vi "Main.vi"() -> ()   [LabVIEW 2013]
uses:
  Ctl/ViewCtl.ctl
  USBCAN/DevType.ctl
  Ctl/DeviceCtl.ctl
  Ctl/ActionCtl.ctl
  Ctl/ResultCtl.ctl
  Ctl/Logctl.ctl
  Ctl/SinResult.ctl
  Global.vi
panel:
  out "Time":u32
  out "Log":refnum<user-event>
  in  "Log":T1
  out "Result":refnum<user-event>
  in  "Result":T2
  in  "输出簇":T3
  in  "设备":T4
  in  "结果显示":T5
  in  "退出":bool
  in  "选项卡控件":enum32{"运行界面", "参数配置", "帮助"}(tab)
  in  "测试方式":enum16{"震动前测试", "震动测试"}(ring)
  in  "设置":bool
  in  "急停":bool
  in  "启动":bool
  out "通信8显示":string
  out "通信7显示":string
  out "通信6显示":string
  out "通信5显示":string
  out "通信4显示":string
  out "通信3显示":string
  out "通信2显示":string
  out "通信1显示":string
  in  "CAN1":bool
  out "CAN1显示":bool
  out "CAN2显示":bool
  in  "CAN2":bool
  out "CAN3显示":bool
  in  "CAN3":bool
  out "CAN4显示":bool
  in  "CAN4":bool
  out "CAN5显示":bool
  in  "CAN5":bool
  out "CAN6显示":bool
  in  "CAN6":bool
  out "CAN7显示":bool
  in  "CAN7":bool
  out "CAN8显示":bool
  in  "CAN8":bool
  out "总结果显示":string
  out "当前模式":string
  in  "COM1":refnum<visa-resource-name>="COM62" caption="COM"
  in  "设备索引1":u16(ring) caption="索引" items=["0", "1", "2", "3", "4", "5", "6", "7"]
  in  "设备索引2":u16(ring)=1 caption="索引" items=["0", "1", "2", "3", "4", "5", "6", "7"]
  in  "COM2":refnum<visa-resource-name>="COM2" caption="COM"
  in  "设备索引3":u16(ring)=2 caption="索引" items=["0", "1", "2", "3", "4", "5", "6", "7"]
  in  "COM3":refnum<visa-resource-name>="COM3" caption="COM"
  in  "设备索引4":u16(ring)=3 caption="索引" items=["0", "1", "2", "3", "4", "5", "6", "7"]
  in  "COM4":refnum<visa-resource-name>="COM4" caption="COM"
  in  "设备索引5":u16(ring)=4 caption="索引" items=["0", "1", "2", "3", "4", "5", "6", "7"]
  in  "COM5":refnum<visa-resource-name>="COM5" caption="COM"
  in  "设备索引6":u16(ring)=5 caption="索引" items=["0", "1", "2", "3", "4", "5", "6", "7"]
  in  "COM6":refnum<visa-resource-name>="COM6" caption="COM"
  in  "设备索引7":u16(ring)=6 caption="索引" items=["0", "1", "2", "3", "4", "5", "6", "7"]
  in  "COM7":refnum<visa-resource-name>="COM7" caption="COM"
  in  "COM8":refnum<visa-resource-name>="COM8" caption="COM"
  in  "设备索引8":u16(ring)=7 caption="索引" items=["0", "1", "2", "3", "4", "5", "6", "7"]
  out "log":string
  out "参数":T7={"帧ID1"=0, "等待延时"=0, "间隔延时"=0, "总时间"=0, "总次数"=0, "发送数据1"="", "接收数据1"="", "发送数据2"="", "接收数据2"="", "CAN盒类型"=3, "帧ID2"=0, "同步启动个数"=8, "模式"=enum."整体", "Baud"=12} {"Baud" items=["250k bps"=10, "10k bps"=2, "5k bps"=1, "50k bps"=5, "40k bps"=4, "20k bps"=3, "80k bps"=6, "100k bps"=7, "125k bps"=8, "200k bps"=9, "400k bps"=11, "500k bps"=12, "666k bps"=13, "800k bps"=14, "1000k bps"=15]; "帧ID2" format="%.0x"; "CAN盒类型" items=["PCI-CAN200"=7, "USB-CAN"=2, "USB-CAN200"=3]; "帧ID1" format="%.0x"}
  # "帧ID\n发送数据域\n接收数据域\n等待延时\n间隔延时\n总次数\n总时间\nCAN盒类型下拉表\n模式：单盒分开测试、整体一起测试 \n布尔显示结果\n布尔开始按钮\n布尔总启动按钮\n过程字符串显示"
  # "ms"
  # "ms"
  # "s"
  # "ms"
  # "ms"
  # "s"
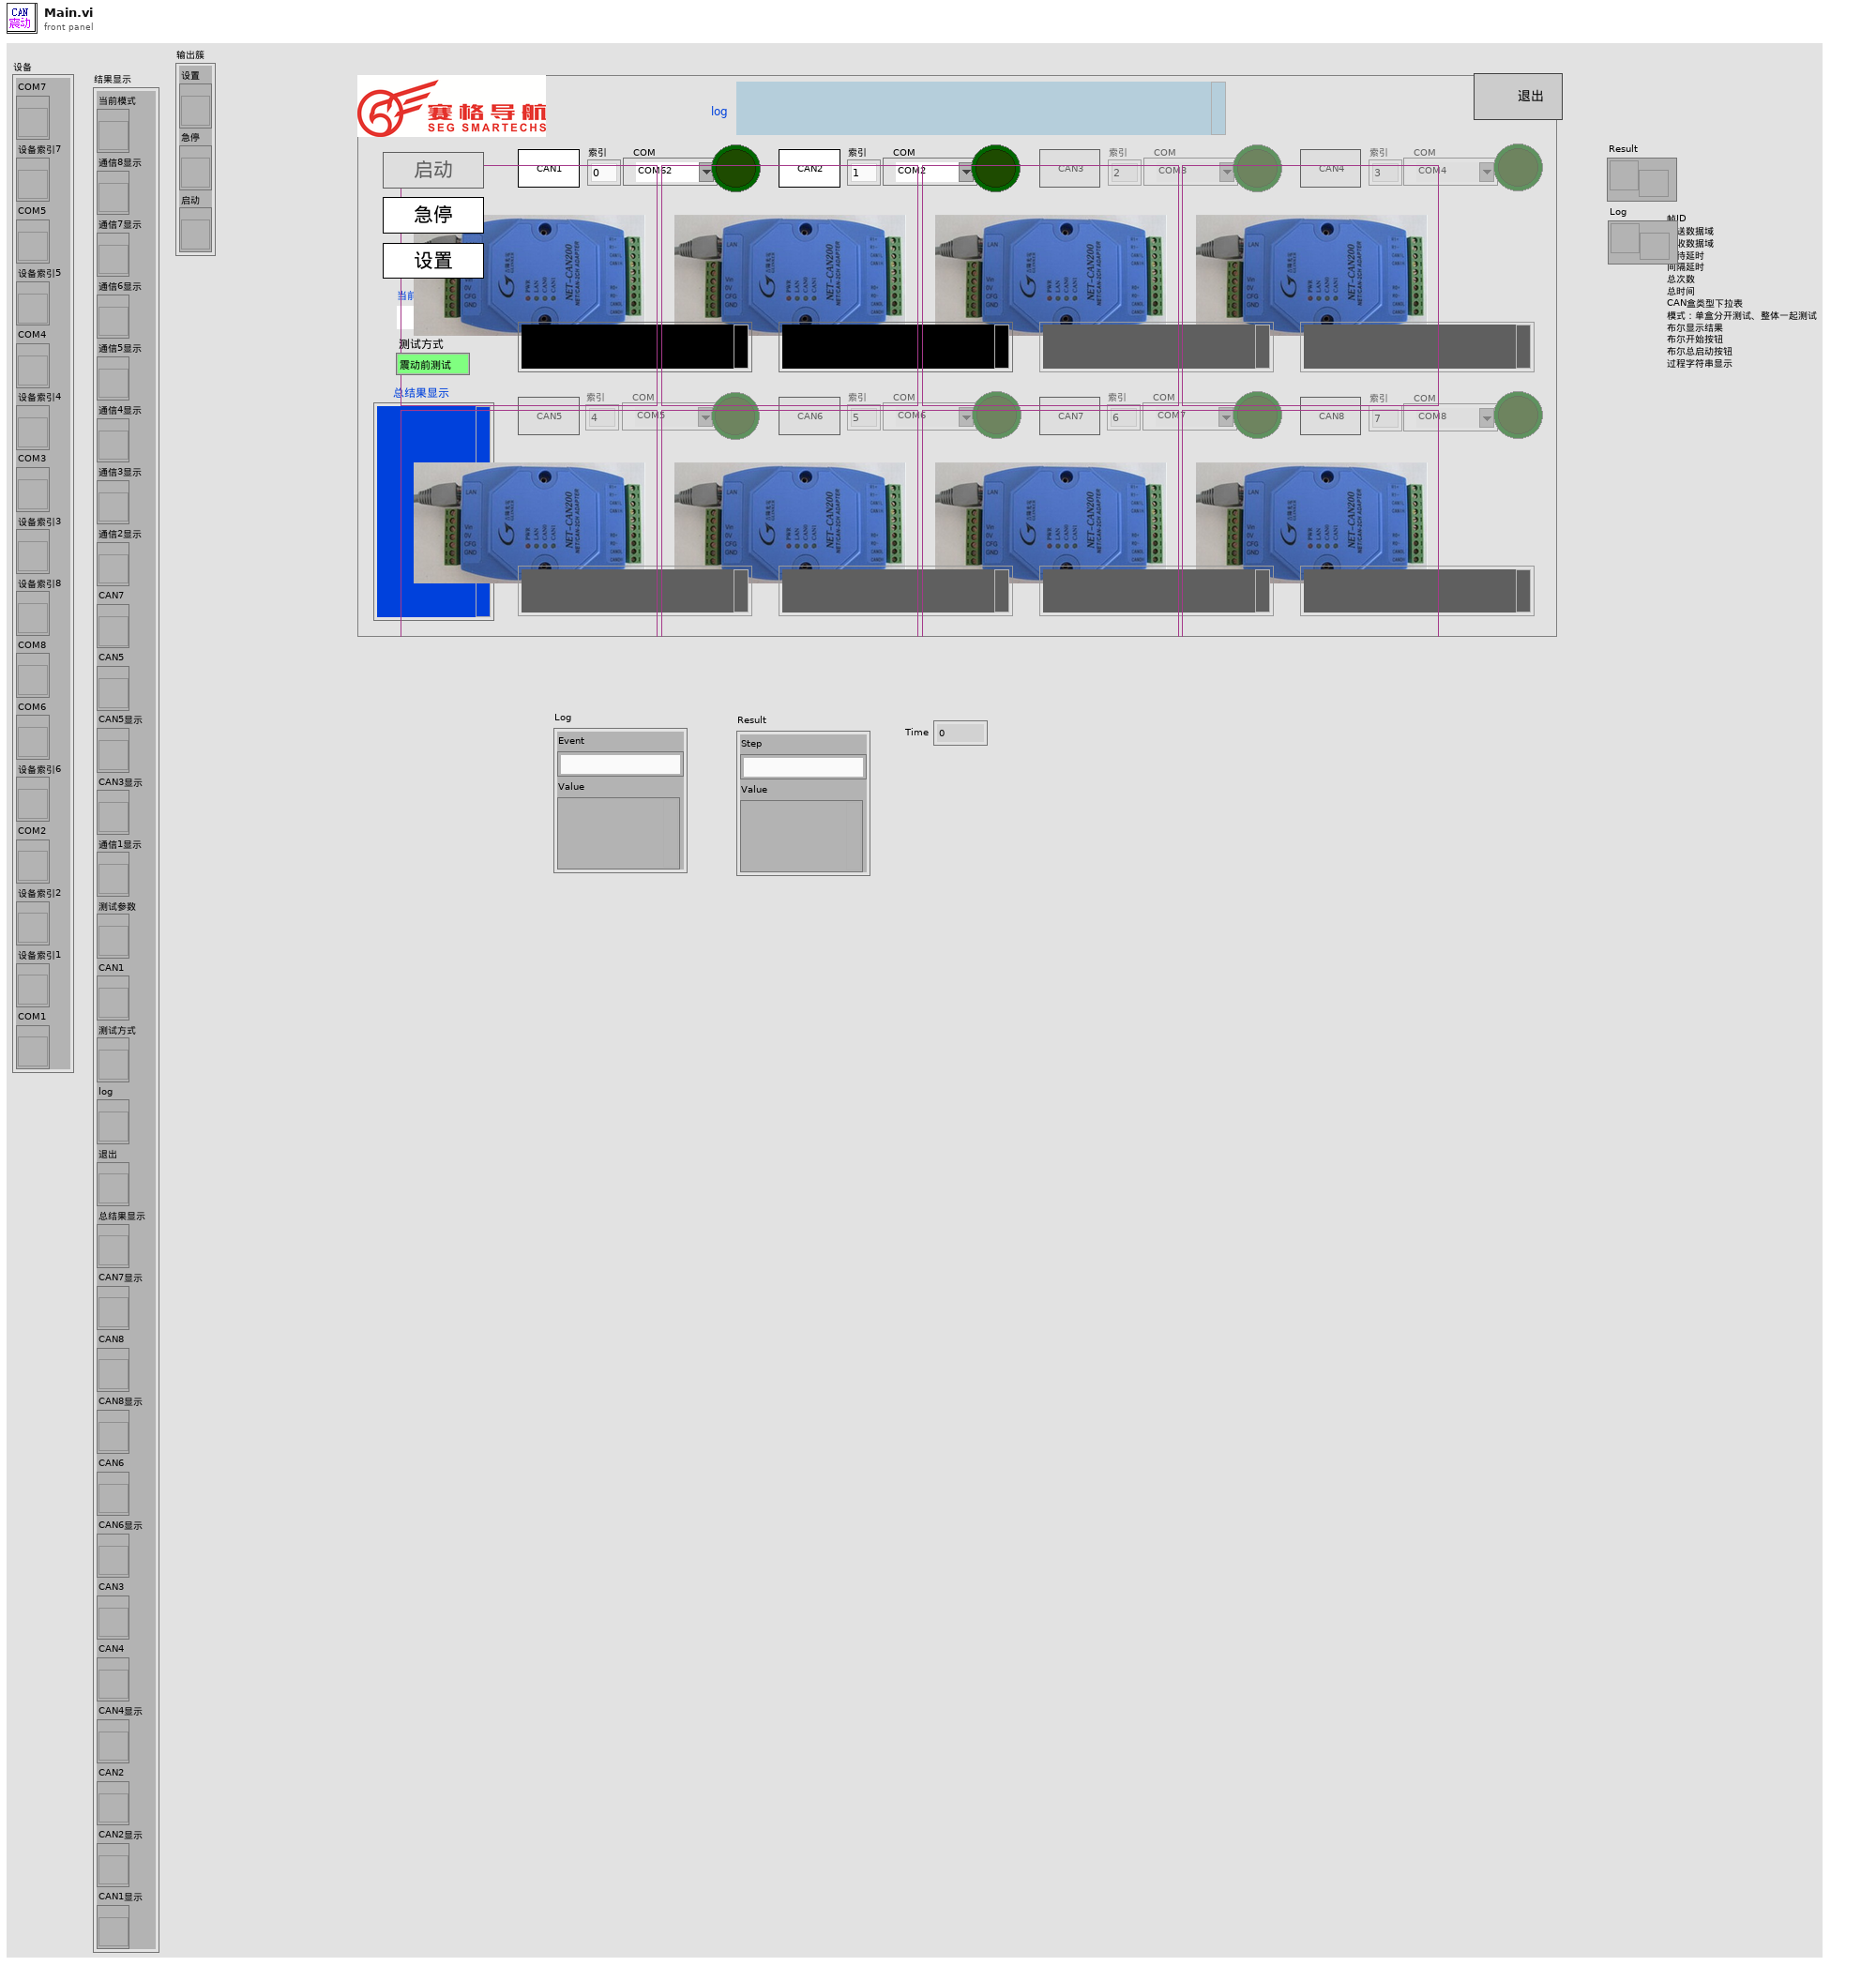
[diagram p1: front panel]
types:
  T1 = typedef "Logctl.ctl" = cluster{"Event":string, "Value":variant}
  T2 = typedef "ResultCtl.ctl" = cluster{"Step":string, "Value":variant}
  T3 = typedef "ActionCtl.ctl" = cluster{"设置":refnum<vi>, "急停":refnum<vi>, "启动":refnum<vi>}
  T4 = typedef "DeviceCtl.ctl" = cluster{"COM7":refnum<vi>, "设备索引7":refnum<vi>, "COM5":refnum<vi>, "设备索引5":refnum<vi>, "COM4":refnum<vi>, "设备索引4":refnum<vi>, "COM3":refnum<vi>, "设备索引3":refnum<vi>, "设备索引8":refnum<vi>, "COM8":refnum<vi>, "COM6":refnum<vi>, "设备索引6":refnum<vi>, "COM2":refnum<vi>, "设备索引2":refnum<vi>, "设备索引1":refnum<vi>, "COM1":refnum<vi>}
  T5 = typedef "ViewCtl.ctl" = cluster{"当前模式":refnum<vi>, "通信8显示":refnum<vi>, "通信7显示":refnum<vi>, "通信6显示":refnum<vi>, "通信5显示":refnum<vi>, "通信4显示":refnum<vi>, "通信3显示":refnum<vi>, "通信2显示":refnum<vi>, "CAN7":refnum<vi>, "CAN5":refnum<vi>, "CAN5显示":refnum<vi>, "CAN3显示":refnum<vi>, "通信1显示":refnum<vi>, "测试参数":refnum<vi>, "CAN1":refnum<vi>, "测试方式":refnum<vi>, "log":refnum<vi>, "退出":refnum<vi>, "总结果显示":refnum<vi>, "CAN7显示":refnum<vi>, "CAN8":refnum<vi>, "CAN8显示":refnum<vi>, "CAN6":refnum<vi>, "CAN6显示":refnum<vi>, "CAN3":refnum<vi>, "CAN4":refnum<vi>, "CAN4显示":refnum<vi>, "CAN2":refnum<vi>, "CAN2显示":refnum<vi>, "CAN1显示":refnum<vi>}
  T6 = typedef "DevType.ctl" = u16
  T7 = cluster{"帧ID1":u32, "等待延时":u32, "间隔延时":u32, "总时间":u32, "总次数":u32, "发送数据1":string, "接收数据1":string, "发送数据2":string, "接收数据2":string, "CAN盒类型":T6, "帧ID2":u32, "同步启动个数":u8, "模式":enum16{"整体", "单个"}, "Baud":u8}
  T8 = enum16{"CAN1", "CAN2", "CAN3", "CAN4", "CAN5", "CAN6", "CAN7", "CAN8"}
  T9 = enum16{"CAN1", "CAN2", "CAN3", "CAN4", "CAN5", "CAN6", "CAN7", "CAN8"}[]
  T10 = cluster{"事件注册引用句柄":refnum<event-registration>, "事件注册引用句柄":refnum<event-registration>}
  T11 = cluster{"COM1":refnum<visa-resource-name>, "COM2":refnum<visa-resource-name>, "COM3":refnum<visa-resource-name>, "COM4":refnum<visa-resource-name>, "COM5":refnum<visa-resource-name>, "COM6":refnum<visa-resource-name>, "COM7":refnum<visa-resource-name>, "COM8":refnum<visa-resource-name>}
  T12 = cluster{"帧ID1":bool, "等待延时":bool, "间隔延时":bool, "总时间":bool, "总次数":bool, "发送数据1":bool, "接收数据1":bool, "发送数据2":bool, "接收数据2":bool, "CAN盒类型":bool, "帧ID2":bool, "同步启动个数":bool, "模式":bool, "Baud":bool}
  T13 = typedef "SinResult.ctl" = cluster{"CAN通道":string, "TsRes":bool}
  T14 = cluster{"kCanBaud":u8, "DeviceType":T6, "DevInd":u16, "间隔延时":u32, "ID1(Hex)":string, "DataIN1(Hex)":string, "DataRec1(Hex)":string, "ID2(Hex)":string, "DataIN2(Hex)":string, "DataRec2(Hex)":string}
  T15 = enum32{"invalid app kind", "Development System", "Run Time System", "Student Edition", "Embedded LabVIEW", "Evaluation", "Custom"}
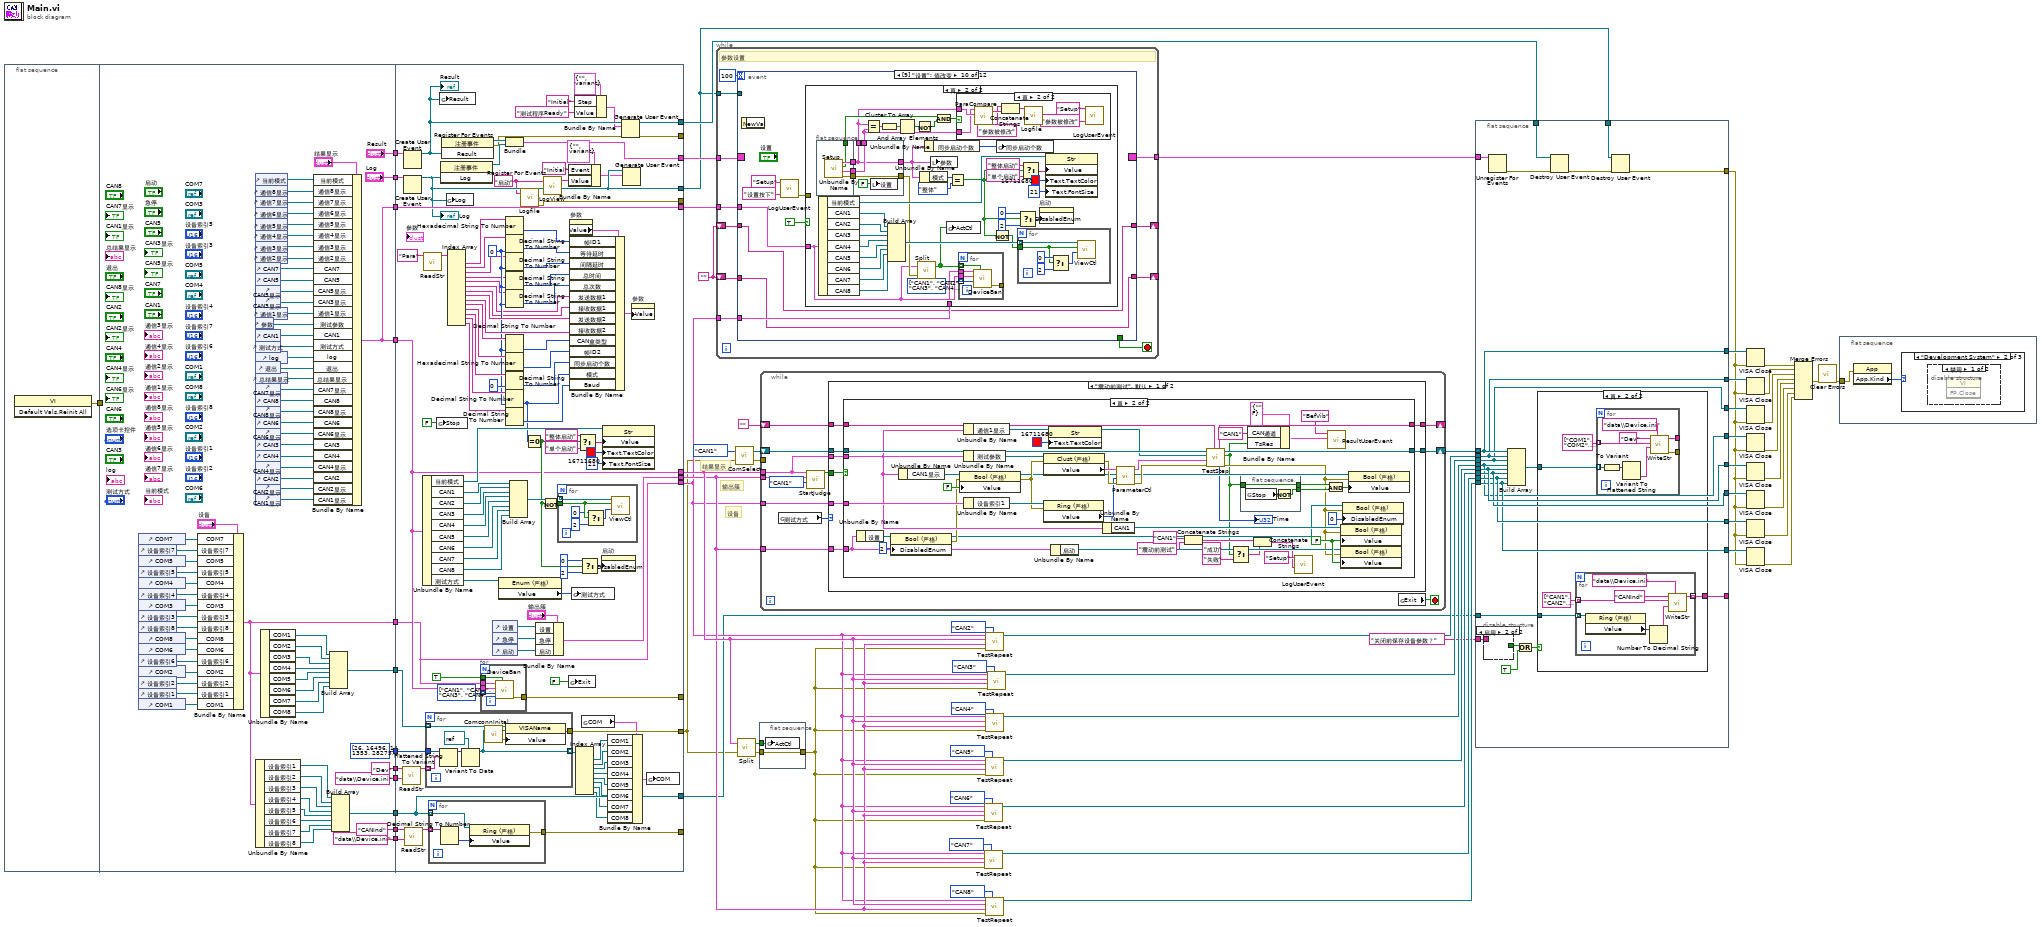
[diagram p0: block diagram]
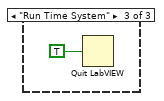
[diagram p4: hidden frame]
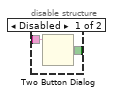
[diagram p5: hidden frame]
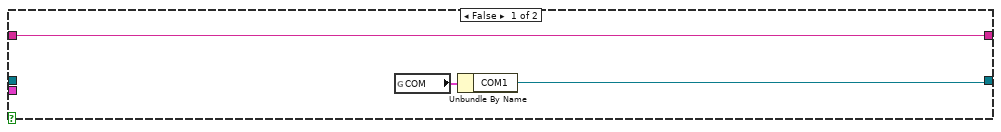
[diagram p7: hidden frame]
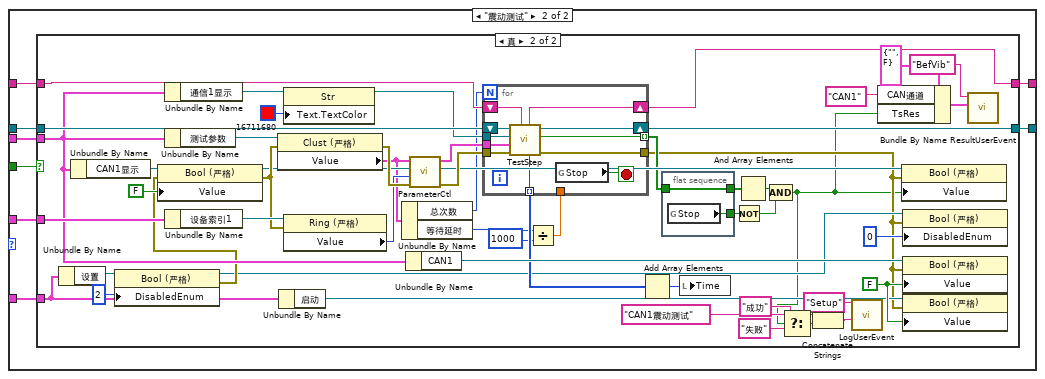
[diagram p8: hidden frame]
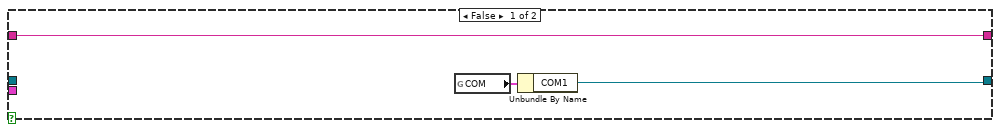
[diagram p9: hidden frame]
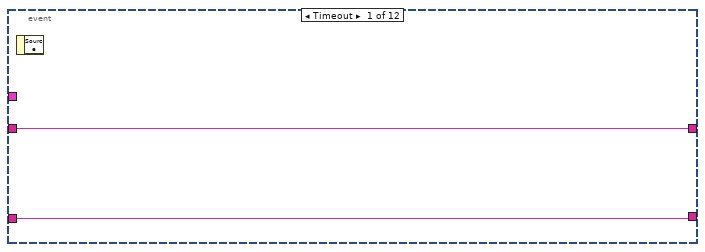
[diagram p10: hidden frame]
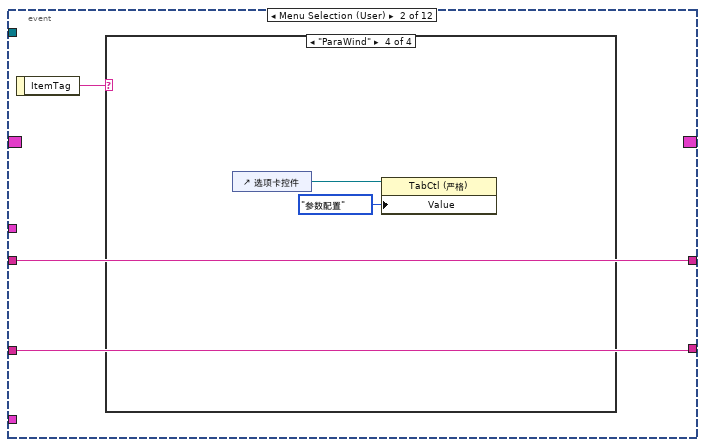
[diagram p11: hidden frame]
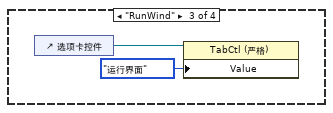
[diagram p14: hidden frame]
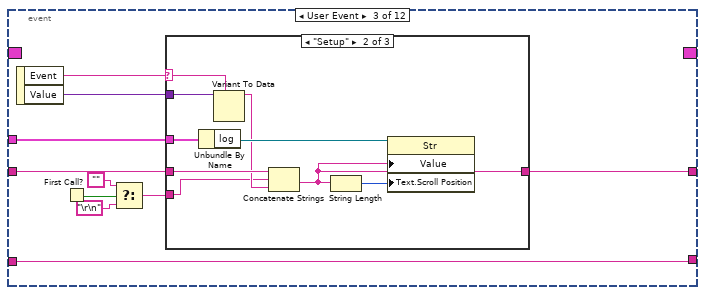
[diagram p15: hidden frame]
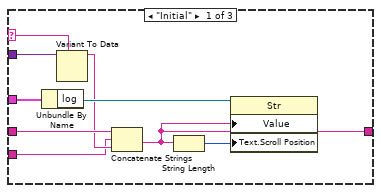
[diagram p16: hidden frame]
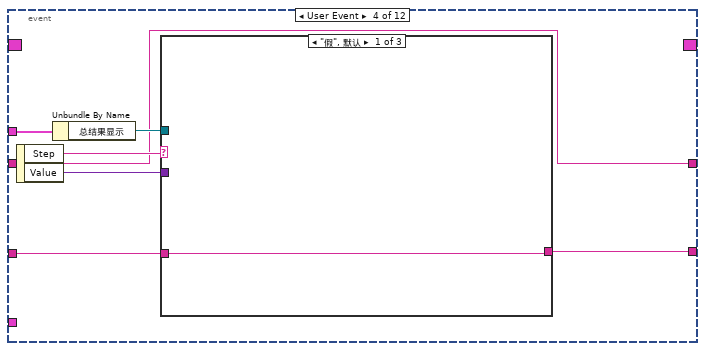
[diagram p18: hidden frame]
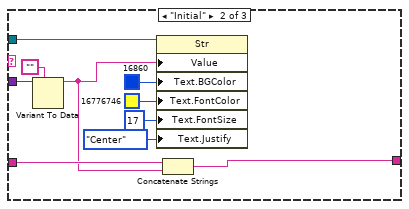
[diagram p19: hidden frame]
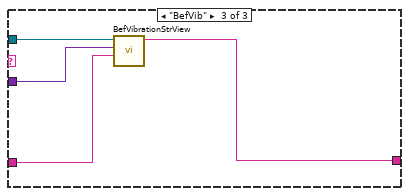
[diagram p20: hidden frame]
diagram:
  w26 = ""
  # "输出簇"
  # "设备"
  # "结果显示"
  n1 = flat-sequence {
    tunnel: [w67] -> w66
    tunnel: w66 -> [_]
    tunnel: [w95] -> w65
    tunnel: [w81] -> w64
    tunnel: [w95] -> w63
    tunnel: ["Dev" ("section")] -> w38
    tunnel: ["data\\Device.ini" ("路径")] -> w37
    tunnel: [i16[] [26, 16496, 14, 1353, 28275, 29810, 3158, 18771, 16855, -13612, -19261, -1101, -14848] ("类型字符串 2")] -> w36
    tunnel: [w82] -> w35
    tunnel: [w72] -> w34
    tunnel: ["CANInd" ("section")] -> w32
    tunnel: ["data\\Device.ini" ("路径")] -> w31
    tunnel: ["Result"] -> w28
    tunnel: ["Log"] -> w27
    tunnel: w65 -> [w187]
    tunnel: w64 -> [w154]
    tunnel: w63 -> [w244]
    tunnel: [w244] -> w62
    tunnel: [w187] -> w60
    tunnel: [w222] -> w59
    tunnel: [w154] -> w58
    tunnel: [w189] -> _
    tunnel: [w183] -> w57
    tunnel: [w176] -> _
    tunnel: [w175] -> w55
    tunnel: [w165] -> w25
    tunnel: w38 -> [w174]
    tunnel: w37 -> [w173]
    tunnel: w36 -> [w172]
    tunnel: w35 -> [w170]
    tunnel: w34 -> [w166]
    tunnel: [w166] -> w33
    tunnel: w32 -> [w169]
    tunnel: w31 -> [w168]
    tunnel: w28 -> [w161]
    tunnel: w27 -> [w160]
    tunnel: [w157] -> _
    tunnel: [w156] -> w12
    tunnel: [w155] -> _
    frame #0 {
      n2 = invoke class="VI" method="Default Vals.Reinit All"() -> (error out=w67:errorcluster)  [unwired: 3 in, 2 out]
    }
    frame #1 {
      n3 = control-ref of="COM7"() -> (w111:refnum<vi>)
      n4 = control-ref of="设备索引7"() -> (w110:refnum<vi>)
      n5 = control-ref of="COM5"() -> (w109:refnum<vi>)
      n6 = control-ref of="设备索引5"() -> (w108:refnum<vi>)
      n7 = control-ref of="COM4"() -> (w107:refnum<vi>)
      n8 = control-ref of="设备索引4"() -> (w106:refnum<vi>)
      n9 = control-ref of="COM3"() -> (w105:refnum<vi>)
      n10 = control-ref of="设备索引3"() -> (w104:refnum<vi>)
      n11 = control-ref of="设备索引8"() -> (w103:refnum<vi>)
      n12 = control-ref of="COM8"() -> (w102:refnum<vi>)
      n13 = control-ref of="COM6"() -> (w101:refnum<vi>)
      n14 = control-ref of="设备索引6"() -> (w100:refnum<vi>)
      n15 = control-ref of="COM2"() -> (w99:refnum<vi>)
      n16 = control-ref of="设备索引2"() -> (w98:refnum<vi>)
      n17 = control-ref of="设备索引1"() -> (w97:refnum<vi>)
      n18 = control-ref of="COM1"() -> (w96:refnum<vi>)
      n19 = Bundle By Name(cluster="设备", "COM7"=w111, "设备索引7"=w110, "COM5"=w109, "设备索引5"=w108, "COM4"=w107, "设备索引4"=w106, "COM3"=w105, "设备索引3"=w104, "设备索引8"=w103, "COM8"=w102, "COM6"=w101, "设备索引6"=w100, "COM2"=w99, "设备索引2"=w98, "设备索引1"=w97, "COM1"=w96) -> (w81:T4)
      n20 = control-ref of="当前模式"() -> (w141:refnum<vi>)
      n21 = control-ref of="通信8显示"() -> (w140:refnum<vi>)
      n22 = control-ref of="通信7显示"() -> (w139:refnum<vi>)
      n23 = control-ref of="通信6显示"() -> (w138:refnum<vi>)
      n24 = control-ref of="通信5显示"() -> (w137:refnum<vi>)
      n25 = control-ref of="通信4显示"() -> (w136:refnum<vi>)
      n26 = control-ref of="通信3显示"() -> (w135:refnum<vi>)
      n27 = control-ref of="通信2显示"() -> (w134:refnum<vi>)
      n28 = control-ref of="CAN7"() -> (w133:refnum<vi>)
      n29 = control-ref of="CAN5"() -> (w132:refnum<vi>)
      n30 = control-ref of="CAN5显示"() -> (w131:refnum<vi>)
      n31 = control-ref of="CAN3显示"() -> (w130:refnum<vi>)
      n32 = control-ref of="通信1显示"() -> (w129:refnum<vi>)
      n33 = control-ref of="参数"() -> (w94:refnum<vi>)
      n34 = control-ref of="CAN1"() -> (w128:refnum<vi>)
      n35 = control-ref of="测试方式"() -> (w127:refnum<vi>)
      n36 = control-ref of="log"() -> (w126:refnum<vi>)
      n37 = control-ref of="退出"() -> (w125:refnum<vi>)
      n38 = control-ref of="总结果显示"() -> (w124:refnum<vi>)
      n39 = control-ref of="CAN7显示"() -> (w123:refnum<vi>)
      n40 = control-ref of="CAN8"() -> (w122:refnum<vi>)
      n41 = control-ref of="CAN8显示"() -> (w121:refnum<vi>)
      n42 = control-ref of="CAN6"() -> (w120:refnum<vi>)
      n43 = control-ref of="CAN6显示"() -> (w119:refnum<vi>)
      n44 = control-ref of="CAN3"() -> (w118:refnum<vi>)
      n45 = control-ref of="CAN4"() -> (w117:refnum<vi>)
      n46 = control-ref of="CAN4显示"() -> (w116:refnum<vi>)
      n47 = control-ref of="CAN2"() -> (w115:refnum<vi>)
      n48 = control-ref of="CAN2显示"() -> (w114:refnum<vi>)
      n49 = control-ref of="CAN1显示"() -> (w113:refnum<vi>)
      n50 = Unbundle By Name(w81) -> ("设备索引1"=w80:refnum<vi>, "设备索引2"=w79:refnum<vi>, "设备索引3"=w78:refnum<vi>, "设备索引4"=w77:refnum<vi>, "设备索引5"=w76:refnum<vi>, "设备索引6"=w75:refnum<vi>, "设备索引7"=w74:refnum<vi>, "设备索引8"=w73:refnum<vi>)
      n51 = Unbundle By Name(w81) -> ("COM1"=w90:refnum<vi>, "COM2"=w89:refnum<vi>, "COM3"=w88:refnum<vi>, "COM4"=w87:refnum<vi>, "COM5"=w86:refnum<vi>, "COM6"=w85:refnum<vi>, "COM7"=w84:refnum<vi>, "COM8"=w83:refnum<vi>)
      n52 = Bundle By Name(cluster="结果显示", "当前模式"=w141, "通信8显示"=w140, "通信7显示"=w139, "通信6显示"=w138, "通信5显示"=w137, "通信4显示"=w136, "通信3显示"=w135, "通信2显示"=w134, "CAN7"=w133, "CAN5"=w132, "CAN5显示"=w131, "CAN3显示"=w130, "通信1显示"=w129, "测试参数"=w94, "CAN1"=w128, "测试方式"=w127, "log"=w126, "退出"=w125, "总结果显示"=w124, "CAN7显示"=w123, "CAN8"=w122, "CAN8显示"=w121, "CAN6"=w120, "CAN6显示"=w119, "CAN3"=w118, "CAN4"=w117, "CAN4显示"=w116, "CAN2"=w115, "CAN2显示"=w114, "CAN1显示"=w113) -> (w95:T5)
      n53 = Build Array(w90, w89, w88, w87, w86, w85, w84, w83) -> (w82:refnum<vi>[])
      n54 = Build Array(w80, w79, w78, w77, w76, w75, w74, w73) -> (w72:refnum<vi>[])
    }
    frame #2 {
      w158 = "启动" ("StrIn")
      w186 = T9 [enum."CAN1", enum."CAN2", enum."CAN3", enum."CAN4", enum."CAN5", enum."CAN6", enum."CAN7", enum."CAN8"] items=["CAN1", "CAN2", "CAN3", "CAN4", "CAN5", "CAN6", "CAN7", "CAN8"]
      w210 = u32 0
      n55 = call "ReadStr.vi"("路径"=w173, "section"=w174) -> ("Value"=w171:string[])  [unwired: 7 in, 2 out]
      n56 = Create User Event(user event datatype=w161) -> (user event=w181:refnum<user-event>)  [unwired: 1 in, 1 out]
      "Result" <- w181
      n57 = Create User Event(user event datatype=w160) -> (user event=w165:refnum<user-event>)  [unwired: 1 in, 1 out]
      "Log" <- w165
      n58 = call "ReadStr.vi"("路径"=w168, "section"=w169) -> ("Value"=w167:string[])  [unwired: 7 in, 2 out]
      n59 = Unbundle By Name(w187) -> ("当前模式"=w243:refnum<vi>, "CAN1"=w240:refnum<vi>, "CAN2"=w239:refnum<vi>, "CAN3"=w238:refnum<vi>, "CAN4"=w237:refnum<vi>, "CAN5"=w236:refnum<vi>, "CAN6"=w235:refnum<vi>, "CAN7"=w234:refnum<vi>, "CAN8"=w233:refnum<vi>, "测试方式"=w228:refnum<vi>)
      n60 = call "ReadStr.vi"("section"="Para") -> ("Value"=w198:string[])  [unwired: 8 in, 2 out]
      n61 = for {
        tunnel: w172 -> [w262]
        tunnel: w171 -> [w261] mode=indexing
        tunnel: w170 -> [w258] mode=indexing
        tunnel: [w257] -> w156
        tunnel: [w254] -> w153 mode=indexing
        n62 = Flattened String To Variant(6:w261, 7:w262) -> (3:w260:variant)  [unwired: 1 in, 1 out]
        n63 = Variant To Data(type=refnum<visa-resource-name> refnum ("VISA资源名称"), Variant=w260) -> (data=w254:refnum<visa-resource-name>)  [unwired: 1 in, 1 out]
        n64 = call "ComconnInital.vi"("COMIn"=w254) -> ("error out"=w256:errorcluster, "COMOut"=w255:refnum<visa-resource-name>)  [unwired: 1 in]
        n65 = property class="VISAName"(reference=w258, error in=w256, "Value"=w255) -> (error out=w257:errorcluster)  [unwired: 1 out]
      }
      n66 = for {
        tunnel: w166 -> [w253] mode=indexing
        tunnel: w167 -> [w252] mode=indexing
        tunnel: [w250] -> w155
        n67 = Decimal String To Number(string=w252) -> (number=w251:i32)  [unwired: 2 in, 1 out]
        n68 = property class="Ring (严格)"(reference=w253, "Value"=w251) -> (error out=w250:errorcluster)  [unwired: 1 in, 1 out]
      }
      n69 = global write "Global.vi" "Stop"(FALSE ("Stop")) -> ()
      n70 = global write "Global.vi" "Result"(w181) -> ()
      n71 = register-events(w165) -> (reference out=w184:refnum<event-registration>)  [unwired: 2 in, 1 out]
      n72 = register-events(w181) -> (reference out=w185:refnum<event-registration>, error out=w182:errorcluster)  [unwired: 2 in]
      n73 = global write "Global.vi" "Log"(w165) -> ()
      n74 = Index Array(array=w198) -> (element #1=w220:string, element #2=w200:string, element #3=w202:string, element #4=w204:string, element #5=w206:string, element #6=w207:string, element #7=w208:string, element #8=w212:string, element #9=w213:string, element #10=w214:string, element #11=w215:string, element #12=w217:string, element #13=w218:string, element #14=w219:string)  [unwired: 14 in]
      n75 = for {
        tunnel: [w267] -> w189
        tunnel: TRUE -> [w266]
        tunnel: w154 -> [w265]
        tunnel: w187 -> [w264]
        tunnel: w186 -> [w263] mode=indexing
        n76 = call "DeviceBan.vi"("Available"=w266, "CAN通路"=w263, "ViewCtl"=w264, "设备"=w265) -> ("error out"=w267:errorcluster)  [unwired: 7 in]
      }
      n77 = control-ref of="设置"() -> (w225:refnum<vi>)
      n78 = control-ref of="急停"() -> (w224:refnum<vi>)
      n79 = control-ref of="启动"() -> (w223:refnum<vi>)
      n80 = property class="Enum (严格)"(reference=w228) -> ("Value"=w227:enum16{"震动前测试", "震动测试"})  [unwired: 1 in, 2 out]
      n81 = Hexadecimal String To Number(string=w220) -> (number=w199:u32)  [unwired: 2 in, 1 out]
      n82 = Decimal String To Number(string=w200, default (0L)=w210) -> (number=w201:u32)  [unwired: 1 in, 1 out]
      n83 = Decimal String To Number(string=w202, default (0L)=w210) -> (number=w203:u32)  [unwired: 1 in, 1 out]
      n84 = Decimal String To Number(string=w204, default (0L)=w210) -> (number=w205:u32)  [unwired: 1 in, 1 out]
      n85 = Decimal String To Number(string=w206, default (0L)=w210) -> (number=w209:u32)  [unwired: 1 in, 1 out]
      n86 = Decimal String To Number(string=w214, default (0L)=w210) -> (number=w216:u32)  [unwired: 1 in, 1 out]
      n87 = Hexadecimal String To Number(string=w215) -> (number=w194:u32)  [unwired: 2 in, 1 out]
      n88 = Decimal String To Number(string=w217, default (0L)=u8 0) -> (number=w193:u8)  [unwired: 1 in, 1 out]
      n89 = Decimal String To Number(string=w218, default (0L)=w210) -> (number=w190:u32)  [unwired: 1 in, 1 out]
      n90 = Decimal String To Number(string=w219) -> (number=w221:i32)  [unwired: 2 in, 1 out]
      n91 = Bundle("事件注册引用句柄"=w185, "事件注册引用句柄"=w184) -> (w183:T10)  [unwired: 1 in]
      n92 = Build Array(w240, w239, w238, w237, w236, w235, w234, w233) -> (w241:refnum<vi>[])
      n93 = call "Logfile.vi"("Data"=w158) -> ("error out"=w157:errorcluster)  [unwired: 10 in]
      n94 = Equal To 0?(x=w190) -> (x = 0?=w229:bool)
      n95 = Bundle By Name(cluster="输出簇", "设置"=w225, "急停"=w224, "启动"=w223) -> (w222:T3)
      n96 = Not(x=w229) -> (.not. x?=w242:bool)
      n97 = call "LogView.vi"("StrIn"=w158) -> ("StrOut"=w159:string)  [unwired: 1 in, 1 out]
      n98 = for {
        tunnel: w241 -> [w272] mode=indexing
        tunnel: w242 -> [w270]
        n99 = Select(t=u32 0, s=w270, f=u32 2) -> (s? t:f=w271:u32)
        n100 = call "ViewCtl.vi"("禁用"=w271, "T？"=w270, "BoolIn"=w272) -> ()  [unwired: 8 in, 1 out]
      }
      n101 = Bundle By Name(cluster=T1 {"Event"="", "Value"=variant} ("Log"), "Event"="Initial" ("Step"), "Value"=w159) -> (w163:T1)
      n102 = global write "Global.vi" "Exit"(FALSE) -> ()
      n103 = property on="参数" class="Clust (严格)"() -> ("Value"=w196:T7)  [unwired: 2 in, 2 out]
      n104 = Bundle By Name(cluster=w196, "帧ID1"=w199, "等待延时"=w201, "间隔延时"=w203, "总时间"=w205, "总次数"=w209, "发送数据1"=w207, "接收数据1"=w208, "发送数据2"=w212, "接收数据2"=w213, "CAN盒类型"=w216, "帧ID2"=w194, "同步启动个数"=w193, "模式"=w190, "Baud"=w221) -> (w195:T7)
      n105 = global write "Global.vi" "测试方式"(w227) -> ()
      n106 = Bundle By Name(cluster=T2 {"Step"="", "Value"=variant} ("Result"), "Step"="Initial", "Value"="测试程序Ready" ("Step")) -> (w179:T2)
      n107 = Index Array(array=w153) -> (element #1=w151:refnum<visa-resource-name>, element #2=w150:refnum<visa-resource-name>, element #3=w149:refnum<visa-resource-name>, element #4=w148:refnum<visa-resource-name>, element #5=w147:refnum<visa-resource-name>, element #6=w146:refnum<visa-resource-name>, element #7=w145:refnum<visa-resource-name>, element #8=w144:refnum<visa-resource-name>)  [unwired: 8 in]
      n108 = Select(t="整体启动", s=w229, f="单个启动") -> (s? t:f=w247:string)
      n109 = Select(t=u32 0, s=w229, f=u32 2) -> (s? t:f=w232:u32)
      n110 = global read "Global.vi" "COM"() -> (w152:T11)
      n111 = property on="启动" class="Bool (严格)"("DisabledEnum"=w232) -> ()  [unwired: 2 in, 2 out]
      n112 = property class="Str"(reference=w243, "Value"=w247, "Text.TextColor"=u32 16711680, "Text.FontSize"=u32 21 ("文本.字体:字号")) -> ()  [unwired: 1 in, 2 out]
      n113 = Bundle By Name(cluster=w152, "COM1"=w151, "COM2"=w150, "COM3"=w149, "COM4"=w148, "COM5"=w147, "COM6"=w146, "COM7"=w145, "COM8"=w144) -> (w143:T11)
      n114 = Generate User Event(user event=w181, event data cluster=w179, error in=w182) -> (user event out=w175:refnum<user-event>, error out=w176:errorcluster)  [unwired: 1 in]
      n115 = Generate User Event(user event=w165, event data cluster=w163) -> ()  [unwired: 2 in, 2 out]
      n116 = property on="参数" class="Clust (严格)"("Value"=w195) -> ()  [unwired: 2 in, 2 out]
      n117 = global write "Global.vi" "COM"(w143) -> ()
    }
  }
  n118 = while {
    tunnel: w62 -> [w281]
    tunnel: w58 -> [w280]
    tunnel: w57 -> [w279]
    shift-right: [w277] -> _
    shift-left: w26 -> [w278]
    tunnel: [w276] -> w56
    shift-right: [w274] -> _
    shift-left: w26 -> [w275]
    tunnel: w25 -> [w273]
    stop <- w283 stop-if-true
    # "参数设置"
    n119 = event shown="[9] \"设置\": 值改变" {
      selector: w279 -> [_ _ _ _ _ _ _ _ _ _ _ _]
      dyn-events: [_ _ _ _ _ _ _ _ _ _ _ _] -> w276
      timeout: 100 -> [_ _ _ _ _ _ _ _ _ _ _ _]
      tunnel: [_ _ _ _ _ _ _ w478 w483 _ _ _] -> w283
      tunnel: w281 -> [_ _ w299 w328 _ _ _ _ _ w496 _ w583]
      tunnel: w280 -> [_ _ _ _ _ _ _ _ _ w495 _ _]
      tunnel: w278 -> [w285 w288 w302 w324 w348 w366 w467 w480 w486 w494 w575 w581]
      tunnel: [w285 w288 w302 w323 w347 w366 w467 w480 w486 w494 w575 w581] -> w277
      tunnel: w275 -> [w284 w287 w298 w322 w346 w364 w466 w479 w485 w492 w574 w580]
      tunnel: [w284 w287 w297 w322 w346 w364 w466 w479 w485 w492 w574 w580] -> w274
      tunnel: w273 -> [_ _ _ _ _ _ _ _ _ _ w569 _]
      event Timeout {
        n120 = event-data() -> ()  [unwired: 1 in, 1 out]
      }
      event Menu Selection (User) {
        n121 = event-data() -> ("ItemTag"=w286:string)  [unwired: 1 in]
        n122 = case shown="\"ParaWind\"" w286 {
          frame "假", Default {
          }
          frame "Help" {
          }
          frame "RunWind" {
            n123 = control-ref of="选项卡控件"() -> (w290:refnum<vi>)
            n124 = property class="TabCtl (严格)"(reference=w290, "Value"=enum32{"运行界面", "参数配置"}."运行界面" ("值")) -> ()  [unwired: 1 in, 2 out]
          }
          frame "ParaWind" {
            n125 = control-ref of="选项卡控件"() -> (w292:refnum<vi>)
            n126 = property class="TabCtl (严格)"(reference=w292, "Value"=enum32{"运行界面", "参数配置"}."参数配置" ("值")) -> ()  [unwired: 1 in, 2 out]
          }
        }
      }
      event User Event {
        n127 = event-data() -> ("Event"=w301:string, "Value"=w300:variant)  [unwired: 1 in]
        n128 = First Call?() -> (First Call?: T/F=w294:bool)
        n129 = Select(t="", s=w294, f="\r\n") -> (s? t:f=w293:string)
        n130 = case shown="\"Setup\"" w301 {
          selector: w301 -> [w310 w319 _]
          tunnel: w300 -> [w311 w320 _]
          tunnel: w299 -> [w309 w318 _]
          tunnel: w298 -> [w307 w316 w321]
          tunnel: [w305 w314 w321] -> w297
          tunnel: w293 -> [w303 w312 _]
          frame "Initial" {
            n131 = Unbundle By Name(w309) -> ("log"=w308:refnum<vi>)
            n132 = Variant To Data(type=w310, Variant=w311) -> (data=w306:string)  [unwired: 1 in, 1 out]
            n133 = Concatenate Strings(w307, w303, w306) -> (w305:string)
            n134 = String Length(string=w305) -> (length=w304:i32)
            n135 = property class="Str"(reference=w308, "Value"=w305, "Text.Scroll Position"=w304) -> ()  [unwired: 1 in, 2 out]
          }
          frame "Setup" {
            n136 = Unbundle By Name(w318) -> ("log"=w317:refnum<vi>)
            n137 = Variant To Data(type=w319, Variant=w320) -> (data=w315:string)  [unwired: 1 in, 1 out]
            n138 = Concatenate Strings(w316, w312, w315) -> (w314:string)
            n139 = String Length(string=w314) -> (length=w313:i32)
            n140 = property class="Str"(reference=w317, "Value"=w314, "Text.Scroll Position"=w313) -> ()  [unwired: 1 in, 2 out]
          }
          frame "真", Default {
          }
        }
      }
      event User Event {
        n141 = event-data() -> ("Step"=w325:string, "Value"=w326:variant)  [unwired: 1 in]
        n142 = Unbundle By Name(w328) -> ("总结果显示"=w327:refnum<vi>)
        n143 = case shown="\"假\", 默认" w325 {
          tunnel: w327 -> [_ w339 w343]
          tunnel: w326 -> [_ w334 w342]
          tunnel: w324 -> [w329 w332 w341]
          tunnel: [w329 w330 w340] -> w323
          frame "假", Default {
          }
          frame "Initial" {
            n144 = Variant To Data(type="", Variant=w334) -> (data=w331:string)  [unwired: 1 in, 1 out]
            n145 = property class="Str"(reference=w339, "Value"=w331, "Text.BGColor"=u32 16860, "Text.FontColor"=u32 16776746, "Text.FontSize"=17, "Text.Justify"=enum16{"Left", "Center", "Right"}."Center" ("文本.调整")) -> ()  [unwired: 1 in, 2 out]
            n146 = Concatenate Strings(w332, w331) -> (w330:string)
          }
          frame "BefVib" {
            n147 = call "BefVibrationStrView.vi"("StrIn"=w341, "Value"=w342, "总结果显示"=w343) -> ("StrOut"=w340:string)  [unwired: 7 in, 1 out]
          }
        }
      }
      event "CAN1", "CAN2", "CAN3", "CAN4", "CAN5", "CAN6", "CAN7", "CAN8", "启动": Value Change {
        n148 = event-data() -> ("CtlRef"=w345:refnum<vi>, "OldVal"=w351:bool, "NewVal"=w349:bool)  [unwired: 1 in]
        n149 = Not(x=w351) -> (.not. x?=w350:bool)
        n150 = And(x=w350, y=w349) -> (x .and. y?=w344:bool)
        n151 = case shown="真" w344 {
          tunnel: w345 -> [_ w353]
          frame False {
          }
          frame True {
            n152 = property class="Bool (严格)"(reference=w353) -> ("Label.Text"=w352:string)  [unwired: 1 in, 2 out]
            n153 = case shown="\"CAN1\", \"CAN2\", \"CAN3\", \"CAN4\", \"CAN5\", \"CAN6\", \"CAN7\", \"CAN8\", \"启动\"" w352 {
              selector: w352 -> [_ w356]
              frame "假", Default {
              }
              frame "CAN1", "CAN2", "CAN3", "CAN4", "CAN5", "CAN6", "CAN7", "CAN8", "启动" {
                n154 = Concatenate Strings(w356, "被按下!" ("字符串")) -> (w354:string)
                n155 = call "LogUserEvent.vi"("StrIn"=w354, "Event"="Setup") -> ()  [unwired: 9 in, 1 out]
              }
            }
          }
        }
        n156 = case shown="假" w344 {
          tunnel: w348 -> [w358 _]
          tunnel: [w358 ""] -> w347
          frame False {
          }
          frame True {
          }
        }
      }
      event "COM2", "COM3", "COM4", "COM5", "COM6", "COM7", "COM8", "COM1": Value Change {
        n157 = event-data() -> ("CtlRef"=w365:refnum<vi>, "OldVal"=w361:refnum<visa-resource-name>, "NewVal"=w360:refnum<visa-resource-name>)  [unwired: 1 in, 2 out]
        n158 = Not Equal?(x=w361, y=w360) -> (x != y?=w362:bool)
        n159 = case shown="真" w362 {
          tunnel: w365 -> [w368 w372]
          tunnel: [w367 w371] -> w363
          tunnel: w361 -> [_ w370]
          tunnel: w360 -> [_ w369]
          frame False {
            n160 = property class="VISAName"(reference=w368) -> ("Label.Text"=w367:string)  [unwired: 1 in, 2 out]
          }
          frame True {
            n161 = property class="VISAName"(reference=w372) -> ("Label.Text"=w371:string)  [unwired: 1 in, 2 out]
            n162 = case shown="\"COM1\", \"COM2\", \"COM3\", \"COM4\", \"COM5\", \"COM6\", \"COM7\", \"COM8\"" w371 {
              selector: w371 -> [_ w380]
              tunnel: w370 -> [_ w378]
              tunnel: w369 -> [_ w377]
              frame "假", Default {
              }
              frame "COM1", "COM2", "COM3", "COM4", "COM5", "COM6", "COM7", "COM8" {
                n163 = call "VariantToStr.vi"("COM"=w378) -> ("ComStr"=w376:string)
                n164 = call "VariantToStr.vi"("COM"=w377) -> ("ComStr"=w374:string)
                n165 = Concatenate Strings(w380, "：值发送改变--原值：", w376, "--新值：", w374) -> (w373:string)
                n166 = call "LogUserEvent.vi"("StrIn"=w373, "Event"="Setup") -> ()  [unwired: 9 in, 1 out]
              }
            }
          }
        }
        n167 = case shown="\"COM1\", 默认" w363 {
          tunnel: w361 -> [w389 w399 w409 w419 w429 w439 w449 w459]
          tunnel: w360 -> [w386 w396 w406 w416 w426 w436 w446 w456]
          frame "COM1", Default {
            n168 = VISA Close(VISA resource name=w389) -> (error out=w387:errorcluster)  [unwired: 1 in]
            n169 = flat-sequence {
              tunnel: 20 -> [w391]
              tunnel: w387 -> [w390]
              tunnel: [w390] -> w385
              frame #0 {
                n170 = Wait (ms)(milliseconds to wait=w391) -> ()  [unwired: 1 out]
              }
            }
            n171 = call "ComconnInital.vi"("error in"=w385, "COMIn"=w386) -> ("COMOut"=w383:refnum<visa-resource-name>)  [unwired: 1 out]
            n172 = global read "Global.vi" "COM"() -> (w384:T11)
            n173 = Bundle By Name(cluster=w384, "COM1"=w383) -> (w382:T11)
            n174 = global write "Global.vi" "COM"(w382) -> ()
          }
          frame "COM2" {
            n175 = VISA Close(VISA resource name=w399) -> (error out=w397:errorcluster)  [unwired: 1 in]
            n176 = flat-sequence {
              tunnel: 20 -> [w401]
              tunnel: w397 -> [w400]
              tunnel: [w400] -> w395
              frame #0 {
                n177 = Wait (ms)(milliseconds to wait=w401) -> ()  [unwired: 1 out]
              }
            }
            n178 = call "ComconnInital.vi"("error in"=w395, "COMIn"=w396) -> ("COMOut"=w393:refnum<visa-resource-name>)  [unwired: 1 out]
            n179 = global read "Global.vi" "COM"() -> (w394:T11)
            n180 = Bundle By Name(cluster=w394, "COM2"=w393) -> (w392:T11)
            n181 = global write "Global.vi" "COM"(w392) -> ()
          }
          frame "COM3" {
            n182 = VISA Close(VISA resource name=w409) -> (error out=w407:errorcluster)  [unwired: 1 in]
            n183 = flat-sequence {
              tunnel: 20 -> [w411]
              tunnel: w407 -> [w410]
              tunnel: [w410] -> w405
              frame #0 {
                n184 = Wait (ms)(milliseconds to wait=w411) -> ()  [unwired: 1 out]
              }
            }
            n185 = call "ComconnInital.vi"("error in"=w405, "COMIn"=w406) -> ("COMOut"=w403:refnum<visa-resource-name>)  [unwired: 1 out]
            n186 = global read "Global.vi" "COM"() -> (w404:T11)
            n187 = Bundle By Name(cluster=w404, "COM3"=w403) -> (w402:T11)
            n188 = global write "Global.vi" "COM"(w402) -> ()
          }
          frame "COM4" {
            n189 = VISA Close(VISA resource name=w419) -> (error out=w417:errorcluster)  [unwired: 1 in]
            n190 = flat-sequence {
              tunnel: 20 -> [w421]
              tunnel: w417 -> [w420]
              tunnel: [w420] -> w415
              frame #0 {
                n191 = Wait (ms)(milliseconds to wait=w421) -> ()  [unwired: 1 out]
              }
            }
            n192 = call "ComconnInital.vi"("error in"=w415, "COMIn"=w416) -> ("COMOut"=w413:refnum<visa-resource-name>)  [unwired: 1 out]
            n193 = global read "Global.vi" "COM"() -> (w414:T11)
            n194 = Bundle By Name(cluster=w414, "COM4"=w413) -> (w412:T11)
            n195 = global write "Global.vi" "COM"(w412) -> ()
          }
          frame "COM5" {
            n196 = VISA Close(VISA resource name=w429) -> (error out=w427:errorcluster)  [unwired: 1 in]
            n197 = flat-sequence {
              tunnel: 20 -> [w431]
              tunnel: w427 -> [w430]
              tunnel: [w430] -> w425
              frame #0 {
                n198 = Wait (ms)(milliseconds to wait=w431) -> ()  [unwired: 1 out]
              }
            }
            n199 = call "ComconnInital.vi"("error in"=w425, "COMIn"=w426) -> ("COMOut"=w423:refnum<visa-resource-name>)  [unwired: 1 out]
            n200 = global read "Global.vi" "COM"() -> (w424:T11)
            n201 = Bundle By Name(cluster=w424, "COM5"=w423) -> (w422:T11)
            n202 = global write "Global.vi" "COM"(w422) -> ()
          }
          frame "COM6" {
            n203 = VISA Close(VISA resource name=w439) -> (error out=w437:errorcluster)  [unwired: 1 in]
            n204 = flat-sequence {
              tunnel: 20 -> [w441]
              tunnel: w437 -> [w440]
              tunnel: [w440] -> w435
              frame #0 {
                n205 = Wait (ms)(milliseconds to wait=w441) -> ()  [unwired: 1 out]
              }
            }
            n206 = call "ComconnInital.vi"("error in"=w435, "COMIn"=w436) -> ("COMOut"=w433:refnum<visa-resource-name>)  [unwired: 1 out]
            n207 = global read "Global.vi" "COM"() -> (w434:T11)
            n208 = Bundle By Name(cluster=w434, "COM6"=w433) -> (w432:T11)
            n209 = global write "Global.vi" "COM"(w432) -> ()
          }
          frame "COM7" {
            n210 = VISA Close(VISA resource name=w449) -> (error out=w447:errorcluster)  [unwired: 1 in]
            n211 = flat-sequence {
              tunnel: 20 -> [w451]
              tunnel: w447 -> [w450]
              tunnel: [w450] -> w445
              frame #0 {
                n212 = Wait (ms)(milliseconds to wait=w451) -> ()  [unwired: 1 out]
              }
            }
            n213 = call "ComconnInital.vi"("error in"=w445, "COMIn"=w446) -> ("COMOut"=w443:refnum<visa-resource-name>)  [unwired: 1 out]
            n214 = global read "Global.vi" "COM"() -> (w444:T11)
            n215 = Bundle By Name(cluster=w444, "COM7"=w443) -> (w442:T11)
            n216 = global write "Global.vi" "COM"(w442) -> ()
          }
          frame "COM8" {
            n217 = VISA Close(VISA resource name=w459) -> (error out=w457:errorcluster)  [unwired: 1 in]
            n218 = flat-sequence {
              tunnel: 20 -> [w461]
              tunnel: w457 -> [w460]
              tunnel: [w460] -> w455
              frame #0 {
                n219 = Wait (ms)(milliseconds to wait=w461) -> ()  [unwired: 1 out]
              }
            }
            n220 = call "ComconnInital.vi"("error in"=w455, "COMIn"=w456) -> ("COMOut"=w453:refnum<visa-resource-name>)  [unwired: 1 out]
            n221 = global read "Global.vi" "COM"() -> (w454:T11)
            n222 = Bundle By Name(cluster=w454, "COM8"=w453) -> (w452:T11)
            n223 = global write "Global.vi" "COM"(w452) -> ()
          }
        }
      }
      event "设备索引1", "设备索引2", "设备索引3", "设备索引4", "设备索引5", "设备索引6", "设备索引7", "设备索引8": Value Change {
        n224 = event-data() -> ("CtlRef"=w465:refnum<vi>, "OldVal"=w464:u16, "NewVal"=w463:u16)  [unwired: 1 in]
        n225 = Not Equal?(x=w464, y=w463) -> (x != y?=w462:bool)
        n226 = case shown="真" w462 {
          tunnel: w465 -> [_ w477]
          tunnel: w464 -> [_ w475]
          tunnel: w463 -> [_ w474]
          frame False {
          }
          frame True {
            n227 = property class="Ring (严格)"(reference=w477) -> ("Label.Text"=w476:string)  [unwired: 1 in, 2 out]
            n228 = Number To Decimal String(number=w475) -> (decimal integer string=w472:string)  [unwired: 1 in]
            n229 = Number To Decimal String(number=w474) -> (decimal integer string=w470:string)  [unwired: 1 in]
            n230 = Concatenate Strings(w476, "：值被修改--原值：", w472, "--新值：", w470) -> (w469:string)
            n231 = call "LogUserEvent.vi"("StrIn"=w469, "Event"="Setup") -> ()  [unwired: 9 in, 1 out]
          }
        }
      }
      event "退出": Value Change {
        n232 = event-data() -> ()  [unwired: 1 in, 1 out]
        n233 = Two Button Dialog(message="程序正在运行，确定退出？" ("消息")) -> (T button?=w478:bool)  [unwired: 2 in]
        n234 = global write "Global.vi" "Exit"(w478) -> ()
        n235 = case shown="真" w478 {
          frame False {
          }
          frame True {
            n236 = call "Logfile.vi"("Data"="退出") -> ()  [unwired: 10 in, 1 out]
          }
        }
      }
      event Panel Close? {
        n237 = event-data() -> ()  [unwired: 1 in, 4 out]
        n238 = Two Button Dialog(message="程序正在运行，确定退出？" ("消息")) -> (T button?=w483:bool)  [unwired: 2 in]
        n239 = global write "Global.vi" "Exit"(w483) -> ()
        n240 = case shown="真" w483 {
          frame False {
          }
          frame True {
            n241 = call "Logfile.vi"("Data"="退出") -> ()  [unwired: 10 in, 1 out]
          }
        }
        n242 = Not(x=w483) -> (.not. x?=w484:bool)
        n243 = event-data("Discard?"=w484) -> ()  [unwired: 1 in, 1 out]
      }
      event "设置": Value Change {
        n244 = event-data() -> ()  [unwired: 1 in, 1 out]
        n245 = call "LogUserEvent.vi"("StrIn"="设置按下", "Event"="Setup") -> ("error out"=w489:errorcluster)  [unwired: 9 in]
        n246 = case shown="真" TRUE {
          tunnel: w496 -> [_ w509]
          tunnel: w495 -> [_ w507]
          tunnel: w489 -> [_ _]
          frame False {
          }
          frame True {
            w508 = T9 [enum."CAN1", enum."CAN2", enum."CAN3", enum."CAN4", enum."CAN5", enum."CAN6", enum."CAN7", enum."CAN8"] items=["CAN1", "CAN2", "CAN3", "CAN4", "CAN5", "CAN6", "CAN7", "CAN8"]
            n247 = flat-sequence {
              tunnel: [w556] -> w536
              tunnel: [w557] -> w535
              tunnel: [w555] -> w506
              tunnel: [w554] -> w505
              tunnel: w536 -> [w558]
              tunnel: [w558] -> w512
              tunnel: w535 -> [w560]
              tunnel: [w560] -> w510
              tunnel: [w559] -> w498
              tunnel: w505 -> [w559]
              tunnel: [w558] -> w499
              frame #0 {
                n248 = call "Setup.vi"() -> ("参数输出"=w556:T7, "Modify?"=w555:bool, "原始参数"=w554:T7, "error out"=w557:errorcluster)  [unwired: 2 in]
              }
              frame #1 {
                n249 = local write "设置"(FALSE) -> ()
              }
            }
            n250 = Unbundle By Name(w509) -> ("当前模式"=w529:refnum<vi>, "CAN1"=w526:refnum<vi>, "CAN2"=w525:refnum<vi>, "CAN3"=w524:refnum<vi>, "CAN4"=w523:refnum<vi>, "CAN5"=w522:refnum<vi>, "CAN6"=w521:refnum<vi>, "CAN7"=w520:refnum<vi>, "CAN8"=w519:refnum<vi>)
            n251 = Equal?(x=w499, y=w498) -> (x = y?=w504:T12)
            n252 = Cluster To Array(cluster=w504) -> (array=w503:bool[])
            n253 = Build Array(w526, w525, w524, w523, w522, w521, w520, w519) -> (w518:refnum<vi>[])
            n254 = And Array Elements(Boolean array=w503) -> (logical AND=w502:bool)
            n255 = Not(x=w502) -> (.not. x?=w501:bool)
            n256 = call "Split.vi"("error in"=w510, "ViewCtl"=w509) -> ("StartArr"=w497:bool[])  [unwired: 1 out]
            n257 = Unbundle By Name(w512) -> ("模式"=w528:enum16{"整体", "单个"})
            n258 = Unbundle By Name(w512) -> ("同步启动个数"=w511:u8)
            n259 = local write "参数"(w512) -> ()
            n260 = And(x=w506, y=w501) -> (x .and. y?=w500:bool)
            n261 = global write "Global.vi" "ActCtl"(w497) -> ()
            n262 = Equal?(x=w528, y=enum16{"整体", "单个"}."整体" ("模式")) -> (x = y?=w513:bool)
            n263 = case shown="真" w500 {
              tunnel: w499 -> [_ w538]
              tunnel: w498 -> [_ w537]
              frame False {
              }
              frame True {
                n264 = call "ParaCompare.vi"("参数输出"=w538, "原始参数"=w537) -> ("StrOut"=w540:string)  [unwired: 8 in, 1 out]
                n265 = Concatenate Strings("参数被修改", w540) -> (w541:string)
                n266 = call "Logfile.vi"("Data"=w541) -> ()  [unwired: 10 in, 1 out]
                n267 = call "LogUserEvent.vi"("StrIn"="参数被修改", "Event"="Setup") -> ()  [unwired: 9 in, 1 out]
              }
            }
            n268 = for {
              tunnel: [w548] -> _
              tunnel: w497 -> [w547] mode=indexing
              tunnel: w507 -> [w546]
              tunnel: w509 -> [w545]
              tunnel: w508 -> [w544] mode=indexing
              n269 = call "DeviceBan.vi"("Available"=w547, "CAN通路"=w544, "ViewCtl"=w545, "设备"=w546) -> ("error out"=w548:errorcluster)  [unwired: 7 in]
            }
            n270 = Not(x=w513) -> (.not. x?=w517:bool)
            n271 = global write "Global.vi" "同步启动个数"(w511) -> ()
            n272 = for {
              tunnel: w518 -> [w553] mode=indexing
              tunnel: w517 -> [w549]
              n273 = Select(t=u32 0, s=w549, f=u32 2) -> (s? t:f=w552:u32)
              n274 = call "ViewCtl.vi"("禁用"=w552, "T？"=w549, "BoolIn"=w553) -> ()  [unwired: 8 in, 1 out]
            }
            n275 = Select(t=u32 0, s=w513, f=u32 2) -> (s? t:f=w514:u32)
            n276 = Select(t="整体启动", s=w513, f="单个启动") -> (s? t:f=w532:string)
            n277 = property on="启动" class="Bool (严格)"("DisabledEnum"=w514) -> ()  [unwired: 2 in, 2 out]
            n278 = property class="Str"(reference=w529, "Value"=w532, "Text.TextColor"=u32 16711680, "Text.FontSize"=u32 21 ("文本.字体:字号")) -> ()  [unwired: 1 in, 2 out]
          }
        }
      }
      event "急停": Value Change {
        n279 = event-data() -> ("OldVal"=w567:bool, "NewVal"=w566:bool)  [unwired: 1 in]
        n280 = Not(x=w567) -> (.not. x?=w568:bool)
        n281 = And(x=w568, y=w566) -> (x .and. y?=w565:bool)
        n282 = case shown="假" w567 {
          tunnel: w566 -> [w576 w578]
          frame False {
            n283 = case shown="真" w576 {
              frame False {
              }
              frame True {
                n284 = global write "Global.vi" "Stop"(TRUE) -> ()
              }
            }
          }
          frame True {
            n285 = case shown="假" w578 {
              frame False {
                n286 = global write "Global.vi" "Stop"(FALSE) -> ()
              }
              frame True {
              }
            }
          }
        }
        n287 = Select(t="急停按下" ("StrIn"), s=w565, f="急停弹起" ("StrIn")) -> (s? t:f=w562:string)
        n288 = call "LogView.vi"("StrIn"=w562) -> ("StrOut"=w573:string)  [unwired: 1 in, 1 out]
        n289 = Bundle By Name(cluster=T1 {"Event"="", "Value"=variant} ("Log"), "Event"="Initial" ("Step"), "Value"=w573) -> (w570:T1)
        n290 = Generate User Event(user event=w569, event data cluster=w570) -> ()  [unwired: 2 in, 2 out]
      }
      event "测试方式": Value Change {
        n291 = event-data() -> ()  [unwired: 1 in, 1 out]
        n292 = Unbundle By Name(w583) -> ("测试方式"=w582:refnum<vi>)
        n293 = property class="Enum (严格)"(reference=w582) -> ("Value"=w584:enum16{"震动前测试", "震动测试"})  [unwired: 1 in, 2 out]
        n294 = global write "Global.vi" "测试方式"(w584) -> ()
      }
    }
  }
  n295 = call "ComSelect.vi"("error in"=w12, "CAN通路"=T8."CAN1") -> ("error out"=w11:errorcluster, "COM1"=w14:refnum<visa-resource-name>)
  n296 = call "Split.vi"("error in"=w12, "ViewCtl"=w60) -> ("error out"=w1:errorcluster, "StartArr"=w10:bool[])
  n297 = flat-sequence {
    tunnel: w10 -> [w586]
    tunnel: [w585] -> w2
    tunnel: w1 -> [w585]
    frame #0 {
      n298 = global write "Global.vi" "ActCtl"(w586) -> ()
    }
  }
  n299 = while {
    tunnel: w60 -> [w591]
    tunnel: w59 -> [w596]
    shift-right: [w592] -> w54
    shift-left: w14 -> [w593]
    tunnel: w58 -> [w590]
    tunnel: w59 -> [w589]
    shift-right: [w587] -> _
    shift-left: "" -> [w588]
    tunnel: w11 -> [_]
    stop <- w598 stop-if-true
    n300 = global read "Global.vi" "测试方式"() -> (w597:enum16{"震动前测试", "震动测试"})
    n301 = call "StartJudge.vi"("CAN通路"=T8."CAN1", "控制簇"=w596, "ParaCtl"=w591) -> ("T/F"=w594:bool)  [unwired: 7 in, 1 out]
    n302 = case shown="\"震动前测试\", 默认" w597 {
      tunnel: w594 -> [w606 w667]
      tunnel: w593 -> [w605 w666]
      tunnel: [w604 w665] -> w592
      tunnel: w591 -> [w603 w664]
      tunnel: w590 -> [w602 w663]
      tunnel: w589 -> [w601 w662]
      tunnel: w588 -> [w600 w661]
      tunnel: [w599 w660] -> w587
      frame "震动前测试", Default {
        n303 = case shown="真" w606 {
          tunnel: w605 -> [_ w656]
          tunnel: [w607 w655] -> w604
          tunnel: w603 -> [_ w631]
          tunnel: w602 -> [_ w649]
          tunnel: w601 -> [_ w624]
          tunnel: w600 -> [w609 w639]
          tunnel: [w609 w638] -> w599
          frame False {
            n304 = global read "Global.vi" "COM"() -> (w608:T11)
            n305 = Unbundle By Name(w608) -> ("COM1"=w607:refnum<visa-resource-name>)
          }
          frame True {
            w641 = FALSE
            n306 = Unbundle By Name(w624) -> ("设置"=w625:refnum<vi>)
            n307 = property class="Bool (严格)"(reference=w625, "DisabledEnum"=2) -> (reference out=w621:refnum<vi>, error out=w622:errorcluster)  [unwired: 1 in]
            n308 = Unbundle By Name(w631) -> ("CAN1显示"=w646:refnum<vi>)
            n309 = property class="Bool (严格)"(reference=w646, error in=w622, "Value"=FALSE) -> (reference out=w643:refnum<vi>, error out=w645:errorcluster)
            n310 = Unbundle By Name(w631) -> ("通信1显示"=w637:refnum<vi>)
            n311 = Unbundle By Name(w631) -> ("测试参数"=w654:refnum<vi>)
            n312 = Unbundle By Name(w649) -> ("设备索引1"=w648:refnum<vi>)
            n313 = property class="Clust (严格)"(reference=w654, error in=w645) -> (error out=w650:errorcluster, "Value"=w653:T7)  [unwired: 1 out]
            n314 = property class="Ring (严格)"(reference=w648, error in=w645) -> ("Value"=w647:u16)  [unwired: 2 out]
            n315 = property class="Str"(reference=w637, "Text.TextColor"=u32 16711680) -> (reference out=w636:refnum<vi>)  [unwired: 1 in, 1 out]
            n316 = Unbundle By Name(w624) -> ("启动"=w640:refnum<vi>)
            n317 = Unbundle By Name(w631) -> ("CAN1"=w642:refnum<vi>)
            n318 = call "ParameterCtl.vi"("error in"=w650, "设备索引"=w647, "参数输入"=w653) -> ("error out"=w651:errorcluster, "输出"=w652:T14)  [unwired: 7 in]
            n319 = Concatenate Strings("CAN1" ("CAN通道"), "震动前测试" ("CAN通道")) -> (w615:string)
            n320 = call "TestStep.vi"("StrInit"=w639, "error in"=w651, "ParaIn"=w652, "ComStr"=w636, "ComIn"=w656) -> ("error out"=w618:errorcluster, "通信？"=w614:bool, "ComOut"=w655:refnum<visa-resource-name>, "Time"=→"Time":u32, "StrOut"=w638:string)  [unwired: 1 in, 1 out]
            n321 = Select(t="成功" ("CAN通道"), s=w614, f="失败" ("CAN通道")) -> (s? t:f=w613:string)
            n322 = flat-sequence {
              tunnel: [w658] -> w633
              tunnel: w614 -> [w657]
              tunnel: [w657] -> w630
              frame #0 {
                n323 = global read "Global.vi" "Stop"() -> (w659:bool)
                n324 = Not(x=w659) -> (.not. x?=w658:bool)
              }
            }
            n325 = Bundle By Name(cluster=T13 {"CAN通道"="", "TsRes"=FALSE} ("CAN结果"), "CAN通道"="CAN1", "TsRes"=w614) -> (w627:T13)
            n326 = Concatenate Strings(w615, w613) -> (w611:string)
            n327 = call "LogUserEvent.vi"("StrIn"=w611, "Event"="Setup") -> ()  [unwired: 9 in, 1 out]
            n328 = And(x=w630, y=w633) -> (x .and. y?=w632:bool)
            n329 = call "ResultUserEvent.vi"("Value"=w627, "Step"="BefVib") -> ()  [unwired: 9 in, 1 out]
            n330 = property class="Bool (严格)"(reference=w642, error in=w618, "Value"=w641) -> ()  [unwired: 2 out]
            n331 = property class="Bool (严格)"(reference=w640, error in=w618, "Value"=w641) -> ()  [unwired: 2 out]
            n332 = property class="Bool (严格)"(reference=w621, error in=w618, "DisabledEnum"=0) -> ()  [unwired: 2 out]
            n333 = property class="Bool (严格)"(reference=w643, error in=w618, "Value"=w632) -> ()  [unwired: 2 out]
          }
        }
      }
      frame "震动测试" {
        n334 = case shown="真" w667 {
          tunnel: w666 -> [_ w722]
          tunnel: [w668 w721] -> w665
          tunnel: w664 -> [_ w697]
          tunnel: w663 -> [_ w716]
          tunnel: w662 -> [_ w684]
          tunnel: w661 -> [w670 w706]
          tunnel: [w670 w705] -> w660
          frame False {
            n335 = global read "Global.vi" "COM"() -> (w669:T11)
            n336 = Unbundle By Name(w669) -> ("COM1"=w668:refnum<visa-resource-name>)
          }
          frame True {
            w708 = FALSE
            n337 = Unbundle By Name(w684) -> ("设置"=w683:refnum<vi>)
            n338 = Unbundle By Name(w697) -> ("CAN1显示"=w713:refnum<vi>)
            n339 = property class="Bool (严格)"(reference=w683, "DisabledEnum"=2) -> (reference out=w680:refnum<vi>, error out=w682:errorcluster)  [unwired: 1 in]
            n340 = property class="Bool (严格)"(reference=w713, error in=w682, "Value"=FALSE) -> (reference out=w710:refnum<vi>, error out=w712:errorcluster)
            n341 = Unbundle By Name(w697) -> ("通信1显示"=w704:refnum<vi>)
            n342 = Unbundle By Name(w697) -> ("测试参数"=w720:refnum<vi>)
            n343 = Unbundle By Name(w716) -> ("设备索引1"=w715:refnum<vi>)
            n344 = property class="Clust (严格)"(reference=w720, error in=w712) -> (error out=w717:errorcluster, "Value"=w701:T7)  [unwired: 1 out]
            n345 = Unbundle By Name(w684) -> ("启动"=w707:refnum<vi>)
            n346 = property class="Str"(reference=w704, "Text.TextColor"=u32 16711680) -> (reference out=w703:refnum<vi>)  [unwired: 1 in, 1 out]
            n347 = property class="Ring (严格)"(reference=w715, error in=w712) -> ("Value"=w714:u16)  [unwired: 2 out]
            n348 = Unbundle By Name(w701) -> ("总次数"=w700:u32, "等待延时"=w686:u32)
            n349 = Unbundle By Name(w697) -> ("CAN1"=w709:refnum<vi>)
            n350 = call "ParameterCtl.vi"("error in"=w717, "设备索引"=w714, "参数输入"=w701) -> ("error out"=w718:errorcluster, "输出"=w719:T14)  [unwired: 7 in]
            n351 = Divide(x=w686, y=1000) -> (x/y=w687:dbl)
            n352 = for {
              N: w700 -> [_]
              tunnel: w719 -> [w733]
              tunnel: w718 -> [w732]
              tunnel: [w725] -> w678
              tunnel: w703 -> [w729]
              tunnel: [w728] -> w695 mode=indexing
              shift-right: [w730] -> w705
              shift-left: w706 -> [w731]
              shift-right: [w734] -> w721
              shift-left: w722 -> [w735]
              tunnel: [w726] -> w689 mode=indexing
              tunnel: w687 -> [_]
              stop <- w727 stop-if-true
              n353 = call "TestStep.vi"("StrInit"=w731, "error in"=w732, "ParaIn"=w733, "ComStr"=w729, "ComIn"=w735) -> ("error out"=w725:errorcluster, "通信？"=w728:bool, "ComOut"=w734:refnum<visa-resource-name>, "Time"=w726:u32, "StrOut"=w730:string)  [unwired: 1 in, 1 out]
              n354 = global read "Global.vi" "Stop"() -> (w727:bool)
            }
            n355 = Add Array Elements(numeric array=w689) -> (sum=w688:u32)
            n356 = flat-sequence {
              tunnel: [w724] -> w699
              tunnel: [w723] -> w696
              tunnel: w695 -> [w723]
              frame #0 {
                n357 = global read "Global.vi" "Stop"() -> (w724:bool)
              }
            }
            n358 = local write "Time"(w688) -> ()
            n359 = Not(x=w699) -> (.not. x?=w698:bool)
            n360 = And Array Elements(Boolean array=w696) -> (logical AND=w691:bool)
            n361 = Compound Arithmetic op=AND(w691, w698) -> (w672:bool)
            n362 = Select(t="成功" ("CAN通道"), s=w672, f="失败" ("CAN通道")) -> (s? t:f=w673:string)
            n363 = Concatenate Strings("CAN1震动测试" ("CAN通道"), w673) -> (w677:string)
            n364 = call "LogUserEvent.vi"("StrIn"=w677, "Event"="Setup") -> ()  [unwired: 9 in, 1 out]
            n365 = Bundle By Name(cluster=T13 {"CAN通道"="", "TsRes"=FALSE} ("CAN结果"), "CAN通道"="CAN1", "TsRes"=w672) -> (w692:T13)
            n366 = property class="Bool (严格)"(reference=w710, error in=w678, "Value"=w672) -> ()  [unwired: 2 out]
            n367 = property class="Bool (严格)"(reference=w680, error in=w678, "DisabledEnum"=0) -> ()  [unwired: 2 out]
            n368 = property class="Bool (严格)"(reference=w709, error in=w678, "Value"=w708) -> ()  [unwired: 2 out]
            n369 = property class="Bool (严格)"(reference=w707, error in=w678, "Value"=w708) -> ()  [unwired: 2 out]
            n370 = call "ResultUserEvent.vi"("Value"=w692, "Step"="BefVib") -> ()  [unwired: 9 in, 1 out]
          }
        }
      }
    }
    n371 = global read "Global.vi" "Exit"() -> (w598:bool)
  }
  n372 = call "TestRepeat.vi"("CAN通路"=T8."CAN7", "error in"=w2, "面板控制"=w59, "结果控制"=w60, "设备"=w58) -> ("ComOut"=w48:refnum<visa-resource-name>)  [unwired: 5 in, 1 out]
  n373 = call "TestRepeat.vi"("CAN通路"=T8."CAN6", "error in"=w2, "面板控制"=w59, "结果控制"=w60, "设备"=w58) -> ("ComOut"=w49:refnum<visa-resource-name>)  [unwired: 5 in, 1 out]
  n374 = call "TestRepeat.vi"("CAN通路"=T8."CAN5", "error in"=w2, "面板控制"=w59, "结果控制"=w60, "设备"=w58) -> ("ComOut"=w50:refnum<visa-resource-name>)  [unwired: 5 in, 1 out]
  n375 = call "TestRepeat.vi"("CAN通路"=T8."CAN8", "error in"=w2, "面板控制"=w59, "结果控制"=w60, "设备"=w58) -> ("ComOut"=w47:refnum<visa-resource-name>)  [unwired: 5 in, 1 out]
  n376 = call "TestRepeat.vi"("CAN通路"=T8."CAN2", "error in"=w2, "面板控制"=w59, "结果控制"=w60, "设备"=w58) -> ("ComOut"=w53:refnum<visa-resource-name>)  [unwired: 5 in, 1 out]
  n377 = call "TestRepeat.vi"("CAN通路"=T8."CAN4", "error in"=w2, "面板控制"=w59, "结果控制"=w60, "设备"=w58) -> ("ComOut"=w51:refnum<visa-resource-name>)  [unwired: 5 in, 1 out]
  n378 = call "TestRepeat.vi"("CAN通路"=T8."CAN3", "error in"=w2, "面板控制"=w59, "结果控制"=w60, "设备"=w58) -> ("ComOut"=w52:refnum<visa-resource-name>)  [unwired: 5 in, 1 out]
  n379 = flat-sequence {
    tunnel: w56 -> [w756]
    tunnel: w55 -> [w753]
    tunnel: w25 -> [w752]
    tunnel: [w751] -> w30
    tunnel: w54 -> [w749]
    tunnel: w53 -> [w748]
    tunnel: w52 -> [w747]
    tunnel: w51 -> [w740]
    tunnel: w50 -> [w746]
    tunnel: w49 -> [w745]
    tunnel: w48 -> [w744]
    tunnel: w47 -> [w743]
    tunnel: [w749] -> w46
    tunnel: [w748] -> w45
    tunnel: [w747] -> w44
    tunnel: [w740] -> w43
    tunnel: [w746] -> w42
    tunnel: [w745] -> w41
    tunnel: [w744] -> w40
    tunnel: [w743] -> w39
    tunnel: w33 -> [w742]
    tunnel: [w741] -> _
    tunnel: "关闭前保存设备参数？" -> [w739]
    frame #0 {
      n380 = disable-structure shown="启用" {
        disable-tunnel: w739 -> [w758 _]
        disable-tunnel: [w757 _] -> w737
        frame Disabled {
          n381 = Two Button Dialog(message=w758) -> (T button?=w757:bool)  [unwired: 2 in]
        }
        frame Enabled {
        }
      }
      n382 = Unregister For Events(event registration refnum=w756) -> (error out=w754:errorcluster)  [unwired: 1 in]
      n383 = Build Array(w749, w748, w747, w740, w746, w745, w744, w743) -> (w750:refnum<visa-resource-name>[])
      n384 = Or(x=w737, y=TRUE) -> (x .or. y?=w736:bool)
      n385 = case shown="真" w736 {
        tunnel: w750 -> [_ w762]
        tunnel: w742 -> [_ w760]
        tunnel: [_ w759] -> w741
        frame False {
        }
        frame True {
          n386 = for {
            tunnel: string[] ["CAN1", "CAN2", "CAN3", "CAN4", "CAN5", "CAN6", "CAN7", "CAN8"] -> [w769] mode=indexing
            tunnel: w760 -> [w767] mode=indexing
            tunnel: [w764] -> w759 mode=indexing
            n387 = property class="Ring (严格)"(reference=w767) -> ("Value"=w766:u16)  [unwired: 1 in, 2 out]
            n388 = Number To Decimal String(number=w766) -> (decimal integer string=w765:string)  [unwired: 1 in]
            n389 = call "WriteStr.vi"("路径"="data\\Device.ini", "value"=w765, "key"=w769, "Section"="CANInd") -> ("ConfigPath"=w764:string)  [unwired: 6 in, 1 out]
          }
          n390 = for {
            tunnel: string[] ["COM1", "COM2", "COM3", "COM4", "COM5", "COM6", "COM7", "COM8"] -> [w777] mode=indexing
            tunnel: w762 -> [w774] mode=indexing
            tunnel: [w772] -> _
            tunnel: [w771] -> _
            n391 = To Variant(anything=w774) -> (Variant=w775:variant)
            n392 = Variant To Flattened String(Variant=w775) -> (data string=w773:string)  [unwired: 1 out]
            n393 = call "WriteStr.vi"("路径"="data\\Device.ini", "value"=w773, "key"=w777, "Section"="Dev") -> ("error out"=w771:errorcluster, "ConfigPath"=w772:string)  [unwired: 6 in]
          }
        }
      }
      n394 = Destroy User Event(user event=w753, error in=w754) -> (error out=w755:errorcluster)
      n395 = Destroy User Event(user event=w752, error in=w755) -> (error out=w751:errorcluster)
    }
  }
  n396 = VISA Close(VISA resource name=w46, error in (no error)=w30) -> (error out=w24:errorcluster)
  n397 = VISA Close(VISA resource name=w45, error in (no error)=w30) -> (error out=w23:errorcluster)
  n398 = VISA Close(VISA resource name=w44, error in (no error)=w30) -> (error out=w22:errorcluster)
  n399 = VISA Close(VISA resource name=w43, error in (no error)=w30) -> (error out=w21:errorcluster)
  n400 = VISA Close(VISA resource name=w42, error in (no error)=w30) -> (error out=w20:errorcluster)
  n401 = VISA Close(VISA resource name=w41, error in (no error)=w30) -> (error out=w19:errorcluster)
  n402 = VISA Close(VISA resource name=w40, error in (no error)=w30) -> (error out=w18:errorcluster)
  n403 = VISA Close(VISA resource name=w39, error in (no error)=w30) -> (error out=w17:errorcluster)
  n404 = Merge Errors(w24, w23, w22, w21, w20, w19, w18, w17) -> (w16:errorcluster)
  n405 = call <vilib>:"Clear Errors.vi"("error in (no error)"=w16) -> ("error out"=w15:errorcluster)  [unwired: 6 in]
  n406 = flat-sequence {
    tunnel: w15 -> [w779]
    frame #0 {
      n407 = property class="App"(error in=w779) -> ("App.Kind"=w780:T15)  [unwired: 1 in, 2 out]
      n408 = case shown="\"Development System\"" w780 {
        frame "invalid app kind", Default {
        }
        frame "Development System" {
          n409 = disable-structure shown="禁用" {
            frame Disabled {
              n410 = invoke class="VI" method="FP.Close"() -> ()  [unwired: 3 in, 3 out]
            }
            frame Enabled {
            }
          }
        }
        frame "Run Time System" {
          n411 = Quit LabVIEW(quit? (T)=TRUE) -> ()
        }
      }
    }
  }
